vi "DialogOnError.vi"(8 "error in (no error)":errorcluster, 10 "Show":bool, 11 "Message":string) -> (0 "error out":errorcluster)   [LabVIEW 2013]
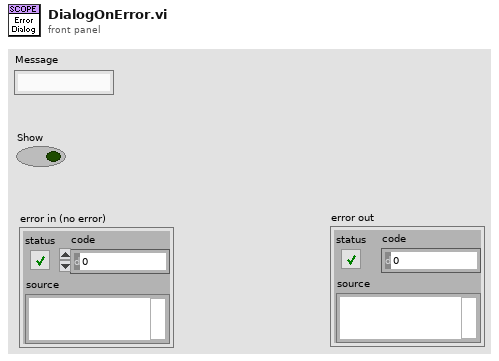
[diagram p1: front panel]
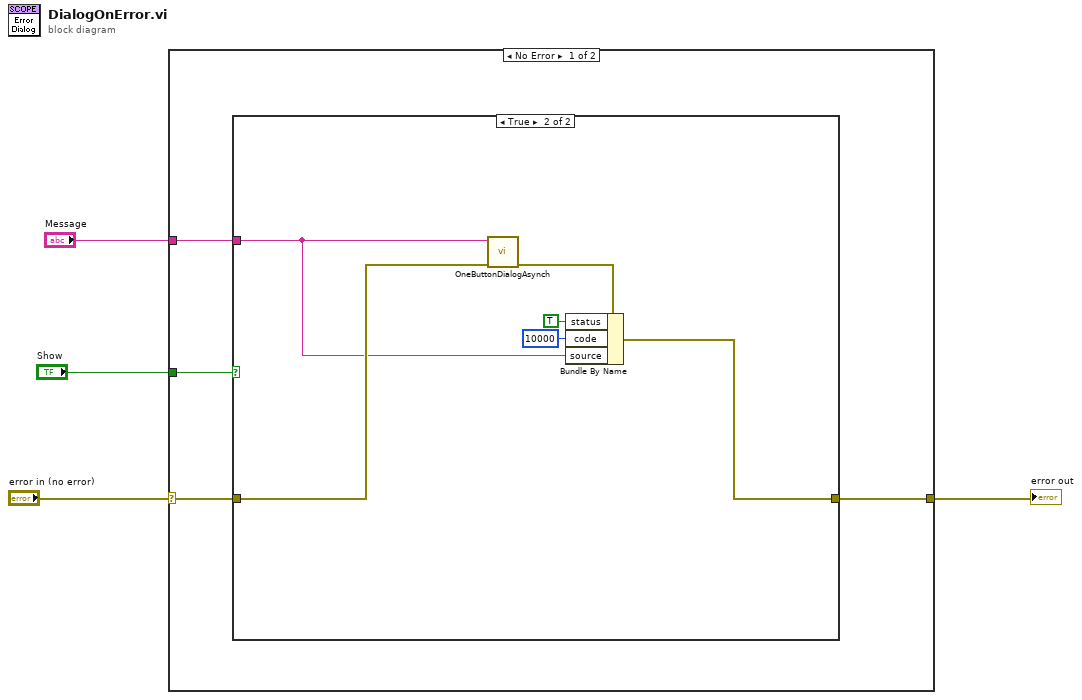
[diagram p0: block diagram]
diagram:
  n1 = case shown="No Error" "error in (no error)" {
    selector: "error in (no error)" -> [w6 w16]
    tunnel: "Show" -> [w8 _]
    tunnel: "Message" -> [w7 _]
    tunnel: [w5 w16] -> w1
    frame No Error {
      n2 = case shown="True" w8 {
        tunnel: w7 -> [_ w11]
        tunnel: w6 -> [w9 w15]
        tunnel: [w9 w10] -> w5
        frame False {
        }
        frame True {
          n3 = call "OneButtonDialogAsynch.vi"("error in (no error)"=w15, "Message to Display"=w11) -> ("error out"=w14:errorcluster)  [unwired: 9 in]
          n4 = Bundle By Name(cluster=w14, "status"=TRUE, "code"=10000, "source"=w11) -> (w10:errorcluster)
        }
      }
    }
    frame Error {
    }
  }
  "error out" <- w1
